vi "ResetStreamingFilter.vi"(8 "error in (no error)":errorcluster, 11 "connection info":T4) -> (0 "error out":errorcluster, 2 "IDs":T1, 3 "connection info":T4)   [LabVIEW 2023, in "J1939 Host Automation API.lvlib"]
uses:
  J1939 Host Automation API.lvlib
  <vilib>/NI/STM/TCP/TCP Connection Info.ctl
  <vilib>/NI/STM/SubVIs/MetaDataElement.ctl
  SubModules/CAN-Streaming-Support/Source/Addon/Addon Shared/Types/Filter Parameters.ctl
  SubModules/CAN-Streaming-Support/Source/Addon/Addon Shared/Types/Direction Filter.ctl
  SubModules/CAN-Streaming-Support/Source/Addon/Addon Shared/Types/Type Filter.ctl
  <vilib>/NI/NI VeriStand Addon Network Comm/Shared/NI VeriStand Addon Network Comm Shared.lvlib
  SubModules/CAN-Streaming-Support/Source/Addon/Addon Shared/CAN Stream Support Shared.lvlib
  <vilib>/NI/STM/NI STM.lvlib
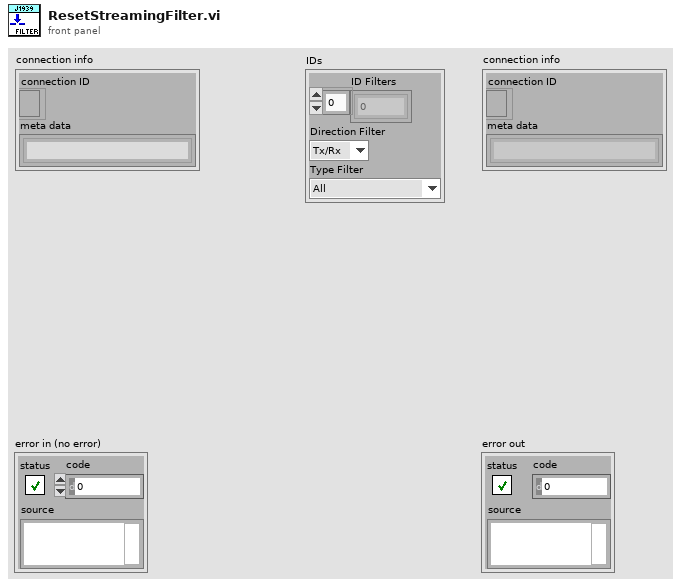
[diagram p1: front panel]
types:
  T1 = typedef "CAN Stream Support Shared.lvlib/Filter Parameters.ctl" = cluster{"ID Filters":u32[], "Direction Filter":T2, "Type Filter":T3}
  T2 = typedef "CAN Stream Support Shared.lvlib/Direction Filter.ctl" = enum16{"Tx/Rx", "Rx", "Tx"}
  T3 = typedef "CAN Stream Support Shared.lvlib/Type Filter.ctl" = enum16{"All", "CAN Data", "CAN Remote", "CAN Bus Error", "CAN 2.0 Data", "CAN FD Data", "CAN FD+BRS Data", "J1939 Data", "Delay", "Log Trigger", "Start Trigger"}
  T4 = typedef "NI STM.lvlib/TCP Connection Info.ctl" = cluster{"connection ID":refnum<k5>, "meta data":T5[]}
  T5 = typedef "NI STM.lvlib/MetaDataElement.ctl" = string
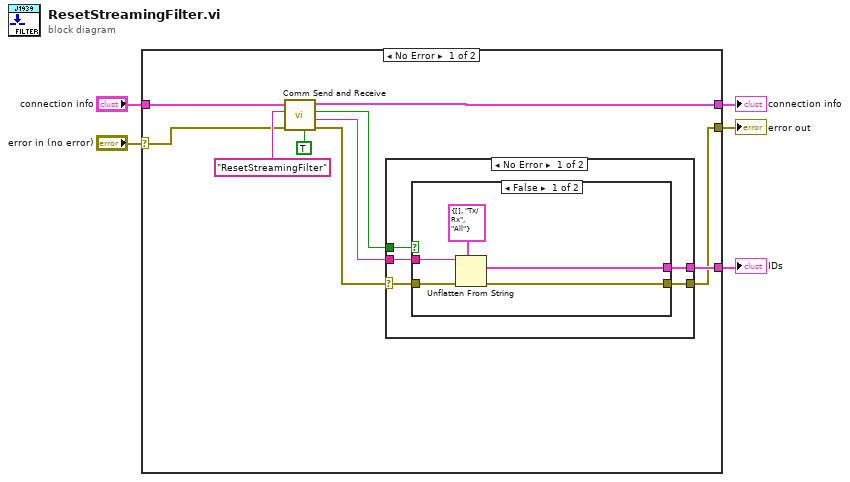
[diagram p0: block diagram]
diagram:
  n1 = case shown="No Error" "error in (no error)" {
    selector: "error in (no error)" -> [w13 w29]
    tunnel: "connection info" -> [w7 w28]
    tunnel: [w6 w28] -> w4
    tunnel: [w8 w29] -> w3
    tunnel: [w10 _] -> w1
    frame No Error {
      n2 = call <vilib>:"Comm Send and Receive.vi"("Resp Required?"=TRUE, "error in (no error)"=w13, "Name"="ResetStreamingFilter", "connection info"=w7) -> ("error out"=w9:errorcluster, "Data"=w11:string, "Timed Out?"=w12:bool, "connection info"=w6:T4)  [unwired: 4 in]
      n3 = case shown="No Error" w9 {
        selector: w9 -> [w18 w27]
        tunnel: w12 -> [w20 _]
        tunnel: [w19 w27] -> w8
        tunnel: w11 -> [w17 _]
        tunnel: [w16 _] -> w10
        frame No Error {
          n4 = case shown="False" w20 {
            tunnel: [w24 w26] -> w19
            tunnel: w18 -> [w25 w26]
            tunnel: w17 -> [w23 _]
            tunnel: [w22 _] -> w16
            frame False {
              n5 = Unflatten From String(type=T1 {"ID Filters"=[], "Direction Filter"=enum."Tx/Rx", "Type Filter"=enum."All"} ("IDs"), binary string=w23, error in (no error)=w25) -> (value=w22:T1, error out=w24:errorcluster)  [unwired: 2 in, 1 out]
            }
            frame True {
            }
          }
        }
        frame Error {
        }
      }
    }
    frame Error {
    }
  }
  "connection info" <- w4
  "error out" <- w3
  "IDs" <- w1
